vi "Get Node Text Content.vi"(8 "error in (no error)":errorcluster, 11 "node in":refnum<k20>) -> (0 "error out":errorcluster, 2 "node text":string, 3 "node out":refnum<k20>)   [LabVIEW 2017, in "Error File Management.lvlib"]
uses:
  Error File Management.lvlib
  <vilib>/xml/Close Reference(Node).vi
  <resource>/objmgr/DOMUserDefRef.rc
  <vilib>/xml/NI_XML.lvlib
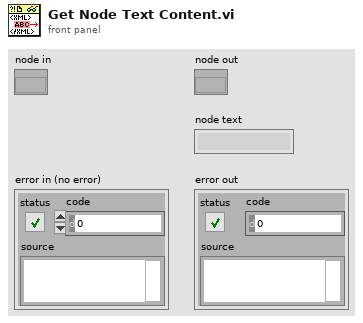
[diagram p1: front panel]
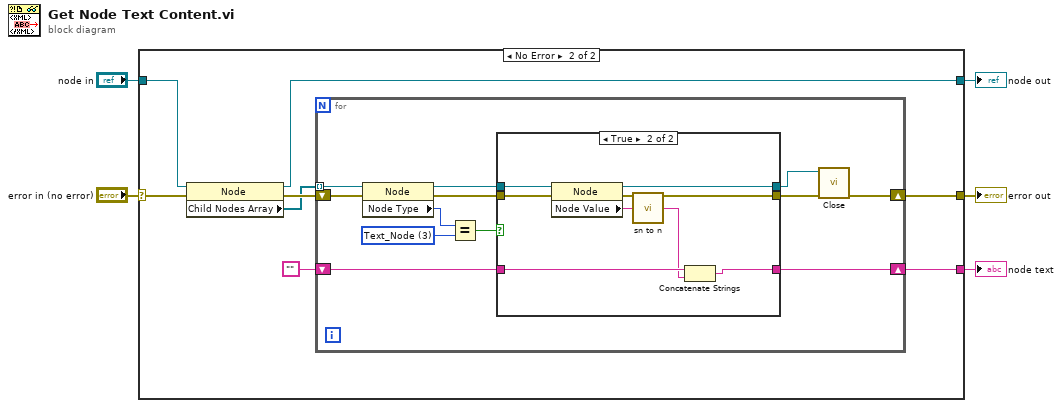
[diagram p0: block diagram]
diagram:
  n1 = case shown="No Error" "error in (no error)" {
    selector: "error in (no error)" -> [w7 w10]
    tunnel: "node in" -> [w6 w15]
    tunnel: [w6 w12] -> w4
    tunnel: [w7 w11] -> w2
    tunnel: [_ w8] -> w1
    frame Error {
    }
    frame No Error {
      n2 = property on="Property Node" class="Node"(reference=w15, error in=w10) -> (reference out=w12:refnum<k20>, error out=w14:errorcluster, "Child Nodes Array"=w13:refnum<k20>[])
      n3 = for {
        shift-right: [w18] -> w11
        shift-left: w14 -> [w26]
        tunnel: w13 -> [w27] mode=indexing
        shift-right: [w16] -> w8
        shift-left: "" -> [w17]
        w24 = 3 items=["Element_Node"=1, "Attribute_Node"=2, "Text_Node"=3, "CDATASection_Node"=4, "EntityReference_Node"=5, "Entity_Node"=6, "ProcessingInstruction_Node"=7, "Comment_Node"=8, "Document_Node"=9, "DocumentType_Node"=10, "DocumentFragment_Node"=11, "Notation_Node"=12] ("Node Type")
        n4 = property class="Node"(reference=w27, error in=w26) -> (reference out=w22:refnum<k20>, error out=w21:errorcluster, "Node Type"=w25:i32)
        n5 = Equal?(x=w25, y=w24) -> (x = y?=w23:bool)
        n6 = case shown="True" w23 {
          tunnel: w22 -> [w30 w38]
          tunnel: w21 -> [w29 w37]
          tunnel: [w30 w36] -> w20
          tunnel: [w29 w32] -> w19
          tunnel: w17 -> [w28 w35]
          tunnel: [w28 w34] -> w16
          frame False {
          }
          frame True {
            n7 = property class="Node"(reference=w38, error in=w37) -> (reference out=w36:refnum<k20>, error out=w32:errorcluster, "Node Value"=w31:string)
            n8 = call "sn to n.vi"("in"=w31) -> ("out"=w33:string)
            n9 = Concatenate Strings(w35, w33) -> (w34:string)
          }
        }
        n10 = call-poly <vilib>:"Close.vi"("error in (no error)"=w19, "node"=w20) -> ("error out"=w18:errorcluster)  [unwired: 7 out]
      }
    }
  }
  "node out" <- w4
  "node text" <- w1
  "error out" <- w2
